vi "Invert Roi.vi"(9 "Invert Columns?":bool, 10 "Invert Roi In":bool[](array[boolean]), 11 "Table Roi In":i32[][](array[numeric])) -> (2 "Invert Roi Out":bool[](array[boolean]), 3 "Table Roi Out":i32[][](array[numeric]))   [LabVIEW 2023]
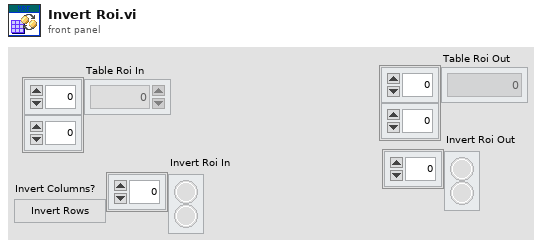
[diagram p1: front panel]
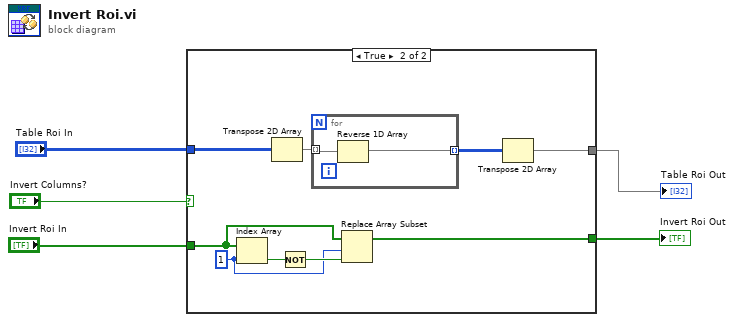
[diagram p0: block diagram]
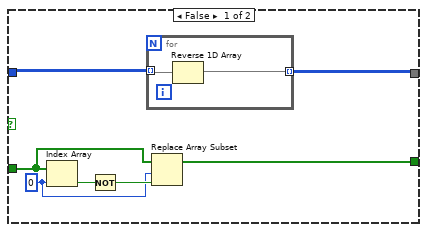
[diagram p2: hidden frame]
diagram:
  n1 = case shown="True" "Invert Columns?" {
    tunnel: [w11 w23] -> w5
    tunnel: "Table Roi In" -> [w12 w20]
    tunnel: "Invert Roi In" -> [w9 w16]
    tunnel: [w6 w15] -> w1
    frame False {
      w7 = 0 ("index")
      n2 = Index Array(array=w9, index=w7) -> (element=w10:bool)
      n3 = Not(x=w10) -> (.not. x?=w8:bool)
      n4 = for {
        tunnel: w12 -> [w14] mode=indexing
        tunnel: [w13] -> w11 mode=indexing
        n5 = Reverse 1D Array(array=w14) -> (reversed array=w13:i32[])
      }
      n6 = Replace Array Subset(array=w9, new element=w8, index=w7) -> (w6:bool[])
    }
    frame True {
      w17 = 1 ("index")
      n7 = Index Array(array=w16, index=w17) -> (element=w19:bool)
      n8 = Transpose 2D Array(2D array=w20) -> (transposed array=w22:i32[][])
      n9 = Not(x=w19) -> (.not. x?=w18:bool)
      n10 = for {
        tunnel: w22 -> [w25] mode=indexing
        tunnel: [w24] -> w21 mode=indexing
        n11 = Reverse 1D Array(array=w25) -> (reversed array=w24:i32[])
      }
      n12 = Replace Array Subset(array=w16, new element=w18, index=w17) -> (w15:bool[])
      n13 = Transpose 2D Array(2D array=w21) -> (transposed array=w23:i32[][])
    }
  }
  "Table Roi Out" <- w5
  "Invert Roi Out" <- w1
